vi "New Verify.vi"(8 "error in":errorcluster, 11 "TestCase in":refnum<class "TestCase.lvclass">) -> (0 "error out":errorcluster, 3 "TestCase out":refnum<class "TestCase.lvclass">)   [LabVIEW 2025, in "VITester.Extension.lvlib"]
uses:
  VITester.Extension.lvlib
  <vilib>/Addons/_JKI Toolkits/VI Tester/TestCase.llb/TestCase.lvclass
  Approval Tests/Options/Options.lvclass/Options.ctl
  Approval Tests/Naming Data/Naming Data.lvclass/Naming Data.ctl
  Approval Tests/Options/Options.lvclass
  Approval Tests/Scrubber/Scrubber.lvclass
  Approval Tests/Namer/Namer.lvclass
  Approval Tests/Naming Data/Naming Data.lvclass
  Approval Tests/Reporter/Reporter.lvclass
  Approval Tests/Text Comparator/Text Comparator.lvclass
  d17fc83f-37f9-40c6-b016-c9b17c74852a.vi
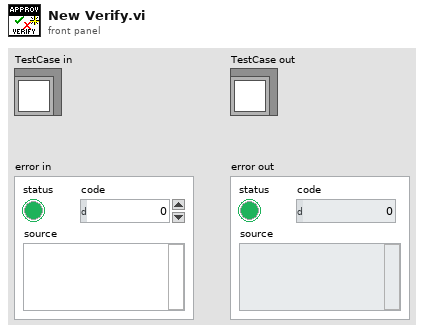
[diagram p1: front panel]
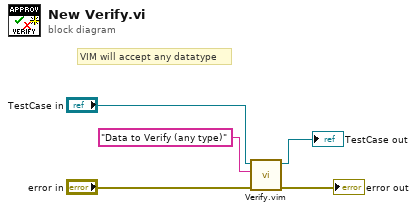
[diagram p0: block diagram]
diagram:
  # "VIM will accept any datatype"
  n1 = call "Verify.vim"("error in"="error in", "Test Data"="Data to Verify (any type)", "TestCase in"="TestCase in") -> ("error out"=→"error out":errorcluster, "TestCase out"=→"TestCase out":refnum<class "TestCase.lvclass">)  [unwired: 7 in]
